vi "DBC Set Signal Value.vi"(7 "Value":dbl, 9 "pSignalName":string, 10 "pMsgName":string, 11 "DBCHandle":u64) -> (1 "pSignalName out":string, 2 "pMsgName out":string, 3 "function return":i32)   [LabVIEW 2010, in "dbc_parser.lvlib"]
doc: "int WINAPI DBC_SetSignalValue(long long DBCHandle, char* pMsgName, char* pSignalName, double Value);"
uses:
  dbc_parser.lvlib
  USB2XXX/trunk/USB2XXX/USB2XXX/vs2019/Release/USB2XXX.dll
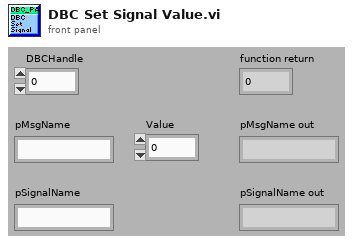
[diagram p1: front panel]
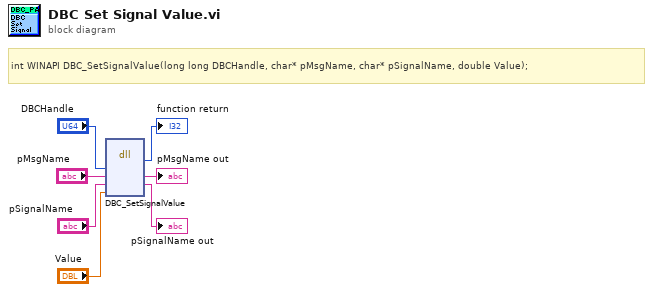
[diagram p0: block diagram]
diagram:
  # "int WINAPI DBC_SetSignalValue(long long DBCHandle, char* pMsgName, char* pSignalName, double Value);"
  n1 = dll-call lib="E:/Projects/USB2XXX/trunk/USB2XXX/USB2XXX/vs2019/Release/USB2XXX.*" fn="DBC_SetSignalValue"("DBCHandle"="DBCHandle", "pMsgName"="pMsgName", "pSignalName"="pSignalName", "Value"="Value") -> (→"function return":i32, "pMsgName"=→"pMsgName out":string, "pSignalName"=→"pSignalName out":string)  [unwired: 5 in, 2 out]
